vi "KeepStatePacketParser.vi"(10 "Message":u8[](array[numeric])) -> ()   [LabVIEW 2014]
panel:
  out "Status":u8
  out "Sequence":u32
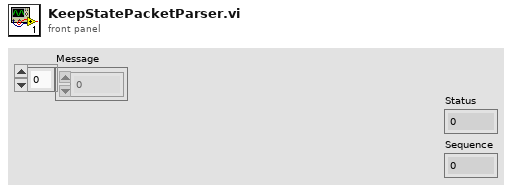
[diagram p1: front panel]
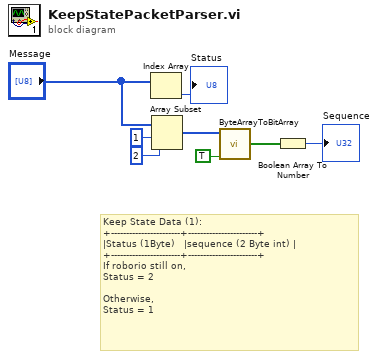
[diagram p0: block diagram]
diagram:
  # "Keep State Data (1):\n+-----------------------+-----------------------+\n|Status (1Byte)\t\t\t|sequence (2 Byte int)\t|\n+-----------------------+-----------------------+\nIf roborio still on,\nStatus = 2\n\nOtherwise,\nStatus = 1"
  n1 = Index Array(array="Message") -> (element=→"Status":u8)  [unwired: 1 in]
  n2 = Array Subset(array="Message", index=1, length=2) -> (w5:u8[])
  n3 = call "ByteArrayToBitArray.vi"("Flip Endian"=TRUE, "Byte Array In"=w5) -> ("Bit Array Out"=w3:bool[])  [unwired: 4 in]
  n4 = Boolean Array To Number(Boolean array=w3) -> (number=→"Sequence":u32)
